vi "EEG read with Filtered PSD Features and classifier with Wii BB FINAL DEMO VERSION.vi"() -> ()   [LabVIEW 2010]
uses:
  <vilib>/Analysis/4window.llb/windowTd.ctl
  <vilib>/Utility/error.llb/DialogType.ctl
  <vilib>/Platform/TimedLoop/XDataNode/XDataNode.xnode
  <vilib>/Platform/TimedLoop/XDataNode/timing_clust.ctl
  <vilib>/Platform/TimedLoop/XDataNode/nitl_modes.ctl
  <vilib>/Platform/TimedLoop/XDataNode/wakeup.ctl
  <vilib>/measure/maspectr.llb/Power Spectrum and PSD Export Mode.ctl
  <vilib>/Analysis/3filter.llb/Filter Passband Type.ctl
  <vilib>/DAQmx/read.llb/DAQmx Read (Analog Wfm 1Chan NSamp).vi
  <vilib>/DAQmx/create/channels.llb/DAQmx Create Channel (AI-Voltage-Basic).vi
  <vilib>/DAQmx/configure/timing.llb/DAQmx Timing (Sample Clock).vi
  <vilib>/Utility/file.llb/Write To Spreadsheet File (DBL).vi
  <vilib>/Analysis/3filter.llb/Butterworth Filter (DBL).vi
  <vilib>/measure/matone.llb/Extract Single Tone Information 1 Chan.vi
  <vilib>/measure/maspectr.llb/FFT Power Spectrum and PSD for 1 Chan.vi
  <vilib>/daqmx/miscellaneous.llb/DAQmx Fill In Error Info.vi
  <vilib>/Waveform/WDTFileIO.llb/Export Waveform To Spreadsheet File.vi
  <vilib>/measure/NI_MAPro.lvlib
  <vilib>/Analysis/NI_AALBase.lvlib
  <vilib>/Analysis/NI_AAL_SigProc.lvlib
  <vilib>/Platform/TimedLoop/XDataNode/XDNodeRunTimeDep.lvlib
  <vilib>/Analysis/NI_AALPro.lvlib
panel:
  in  "input terminal configuration":i32(ring)=-1 items=["default"=-1, "RSE"=10083, "NRSE"=10078, "Differential"=10106, "Pseudodifferential"=12529]
  in  "Save Wii BB":bool
  in  "stop 2":bool
  in  "index":i32
  out "Button":bool
  out "X":dbl
  out "Y":dbl
  in  "LED":bool
  out "error out":errorcluster
  out "XY Balance Board":cluster{dbl[], dbl[]}(graph)
  in  "Low Cutoff Frequency":dbl(slide) scale=0.0..100.0
  in  "High Cutoff Frequency":dbl(slide) scale=0.0..500.0
  in  "String to be appended in filename":string
  in  "Slide":dbl(slide) scale=0.0..0.0005
  in  "WINDOW":T1=1 items=["Rectangle"=0, "Hanning"=1, "Hamming"=2, "Blackman-Harris"=3, "Exact Blackman"=4, "Blackman"=5, "Flat Top"=6, "4 Term B-Harris "=7, "7 Term B-Harris"=8, "Low Sidelobe"=9, "Blackman Nuttall"=11, "Triangle"=30, "Bartlett-Hanning"=31, "Bohman"=32, "Parzen"=33, "Welch"=34, "Kaiser"=60, "Dolph-Chebyshev"=61, "Gaussian"=62]
  out "Amplitudes":dbl[](array[numeric])
  out "FREQUENCY":dbl[](array[numeric])
  in  "Min. No. of Peaks\n to be detected":i32
  out "# found":i32
  out "BRAIN SWITCH":bool
  out "PSD Filtered Waveform":cluster{"f0":dbl, "df":dbl, "magnitude":dbl[]}(graph)
  in  "Path":path
  in  "SAVE TO FILE":bool
  out "new file path (Not A Path if cancelled)":path
  out "df":dbl
  out "magnitude":dbl[](array[numeric])
  out "f0":dbl
  in  "PARAMETERS":T2={"averaging mode"=enum."No averaging", "weighting mode"=enum."Linear", "number of averages"=10}
  out "Test SIGNAL AMPLITUDE":dbl format="%.2p"
  out "Test SIGNAL FREQUENCY":dbl format="%.2p"
  in  "BUFFER SIZE":dbl
  out "FILTERED Waveform Graph":waveform(dbl)(graph)
  in  "stop":bool
  in  "SAMPLE RATE":dbl=1000.0 format="%0.2f"
  # "EEG DATA ACQUISITION AND ANALYSIS"
  # "DAQ PARAMETERS"
  # "FEATURES EXTRACTED"
  # "BAND PASS FILTER CHARACTERSTICS"
  # "AVERAGING PARAMETERS and FEATURES EXTRACTED FROM THE FILTERED PSD"
  # "Wii BB CONTROLS and INDICATORS"
  # "THRESHOLD CLASSIFIER"
  # "FILE SAVING MODULE"
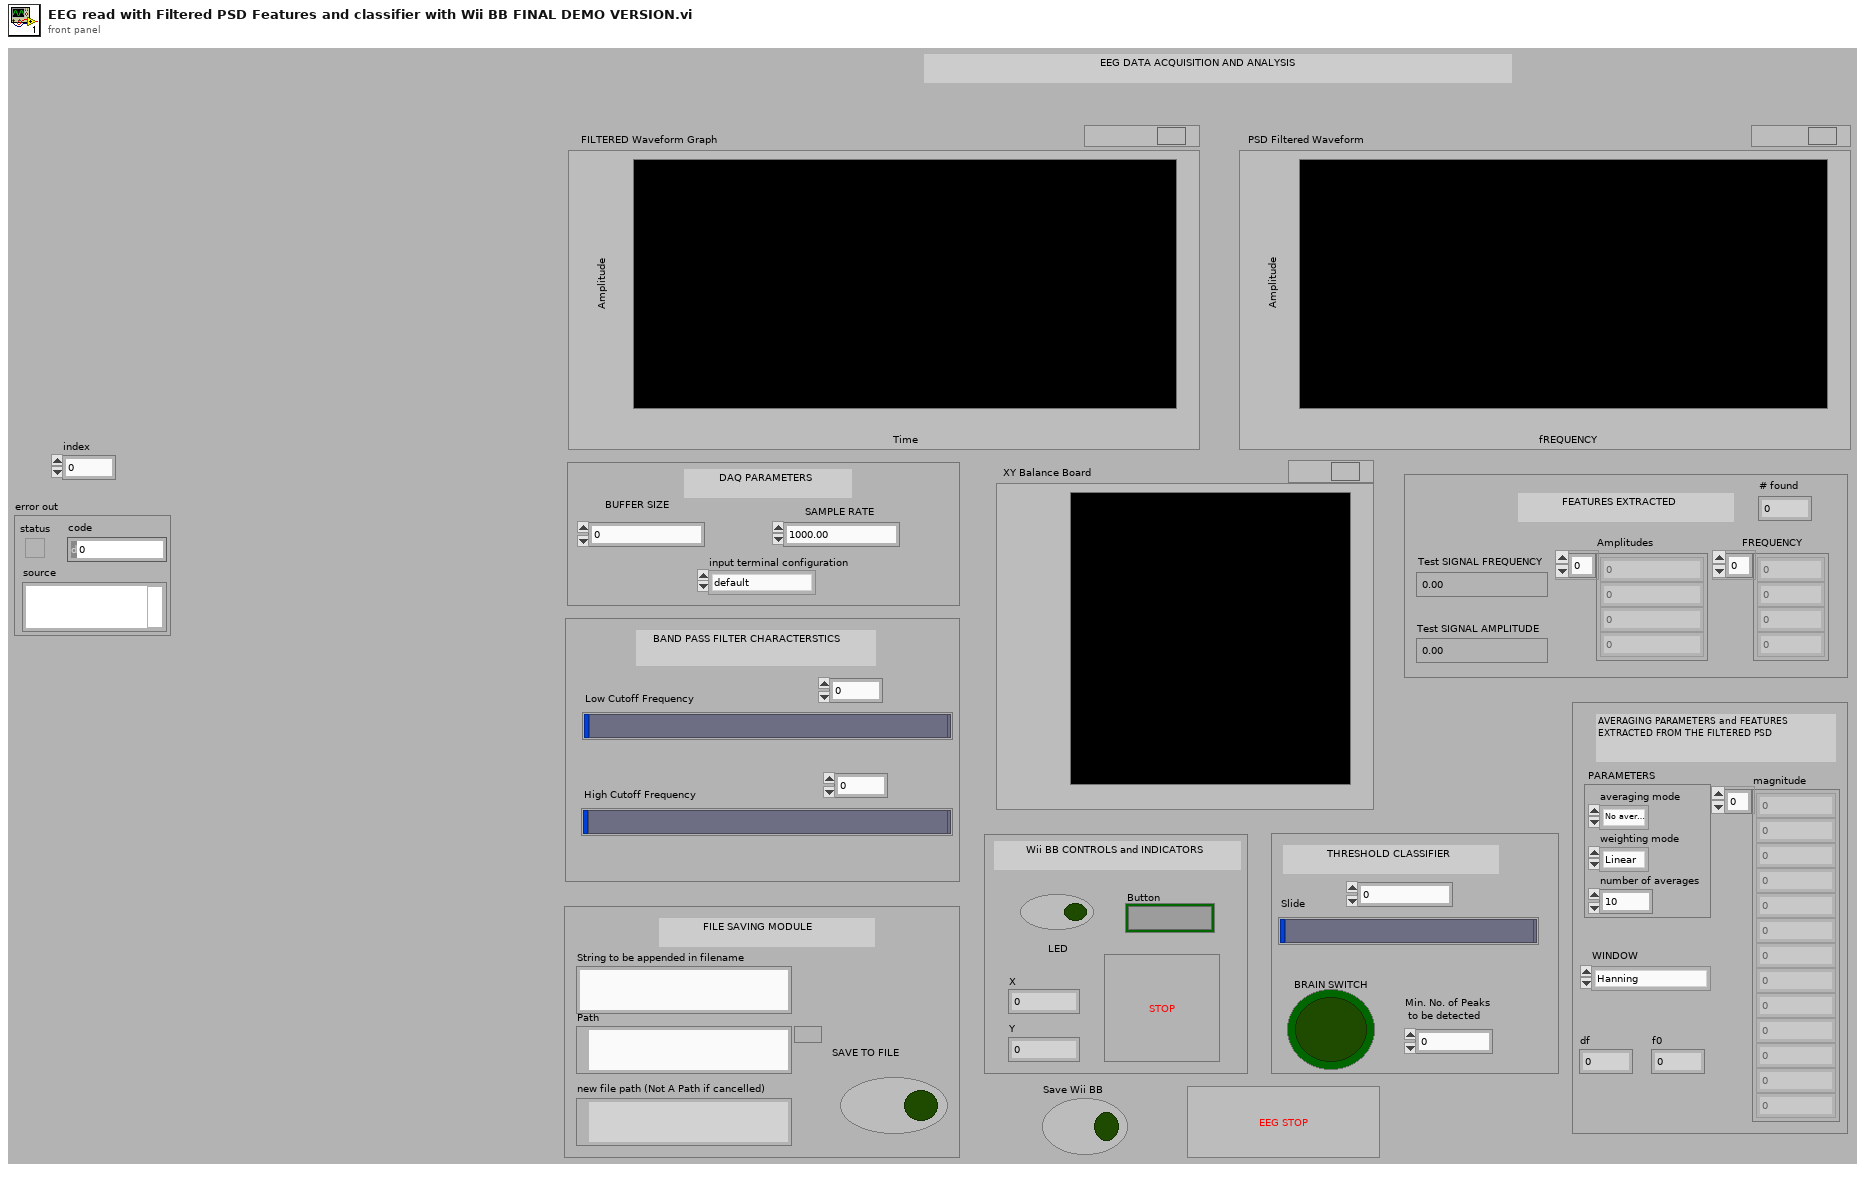
[diagram p1: front panel]
types:
  T1 = typedef "NI_AALPro.lvlib/windowTd.ctl" = u32
  T2 = cluster{"averaging mode":enum16{"No averaging", "Vector averaging", "RMS averaging", "Peak hold"}, "weighting mode":enum16{"Linear", "Exponential"}, "number of averages":u32}
  T3 = typedef "DialogType.ctl" = u16
  T4 = cluster{"right-top zero":i16, "right-bottom zero":i16, "left-top zero":i16, "left-bottom zero":i16}
  T5 = cluster{"Right-top":i16, "Right-bottom":i16, "Left-top":i16, "Left-bottom":i16, "X":dbl, "Y":dbl, "Sum":dbl}
  T6 = typedef "NI_Matrix.lvlib/RealMatrix.ctl" = dbl[][]
  T7 = typedef "XDNodeRunTimeDep.lvlib/timing_clust.ctl" = cluster{"Expected End [f-1]":u64, "Actual End [f-1]":u64, "Finished Late? [f-1]":bool, "Expected End [i-1]":u64, "Actual End [i-1]":u64, "Finished Late? [i-1]":bool, "Expected Start [i]":u64, "Actual Start [i]":u64, "Expected Start [f]":u64, "Actual Start [f]":u64, "Source Name":string, "Structure Name":string, "Period":i64, "Deadline":i64, "Offset":i64, "Start":i64, "Priority":i32, "Timeout":i32, "Mode":T8, "Wakeup Reason":T9, "Error":errorcluster, "Source Type":string, "Secondary Source Type":string, "Global End Time":u64, "Global Start Time":u64, "Frame Duration":u64, "Iteration Duration":u64, "Assigned CPU":i32, "I/O Scan Engine Mode":u32}
  T8 = typedef "XDNodeRunTimeDep.lvlib/nitl_modes.ctl" = enum32{"No Change", "Process missed periods, maintain original phase", "Discard missed periods, maintain original phase", "Process missed periods, ignore original phase", "Discard missed periods, ignore original phase"}
  T9 = typedef "XDNodeRunTimeDep.lvlib/wakeup.ctl" = enum32{"Normal", "Aborted", "Asynchronous wakeup", "Timing source error", "Timed loop error", "Timeout"}
  T10 = typedef "NI_AALBase.lvlib/Filter Passband Type.ctl" = enum32{"Lowpass", "Highpass", "Bandpass", "Bandstop"}
  T11 = typedef "NI_MAPro.lvlib/Power Spectrum and PSD Export Mode.ctl" = u16
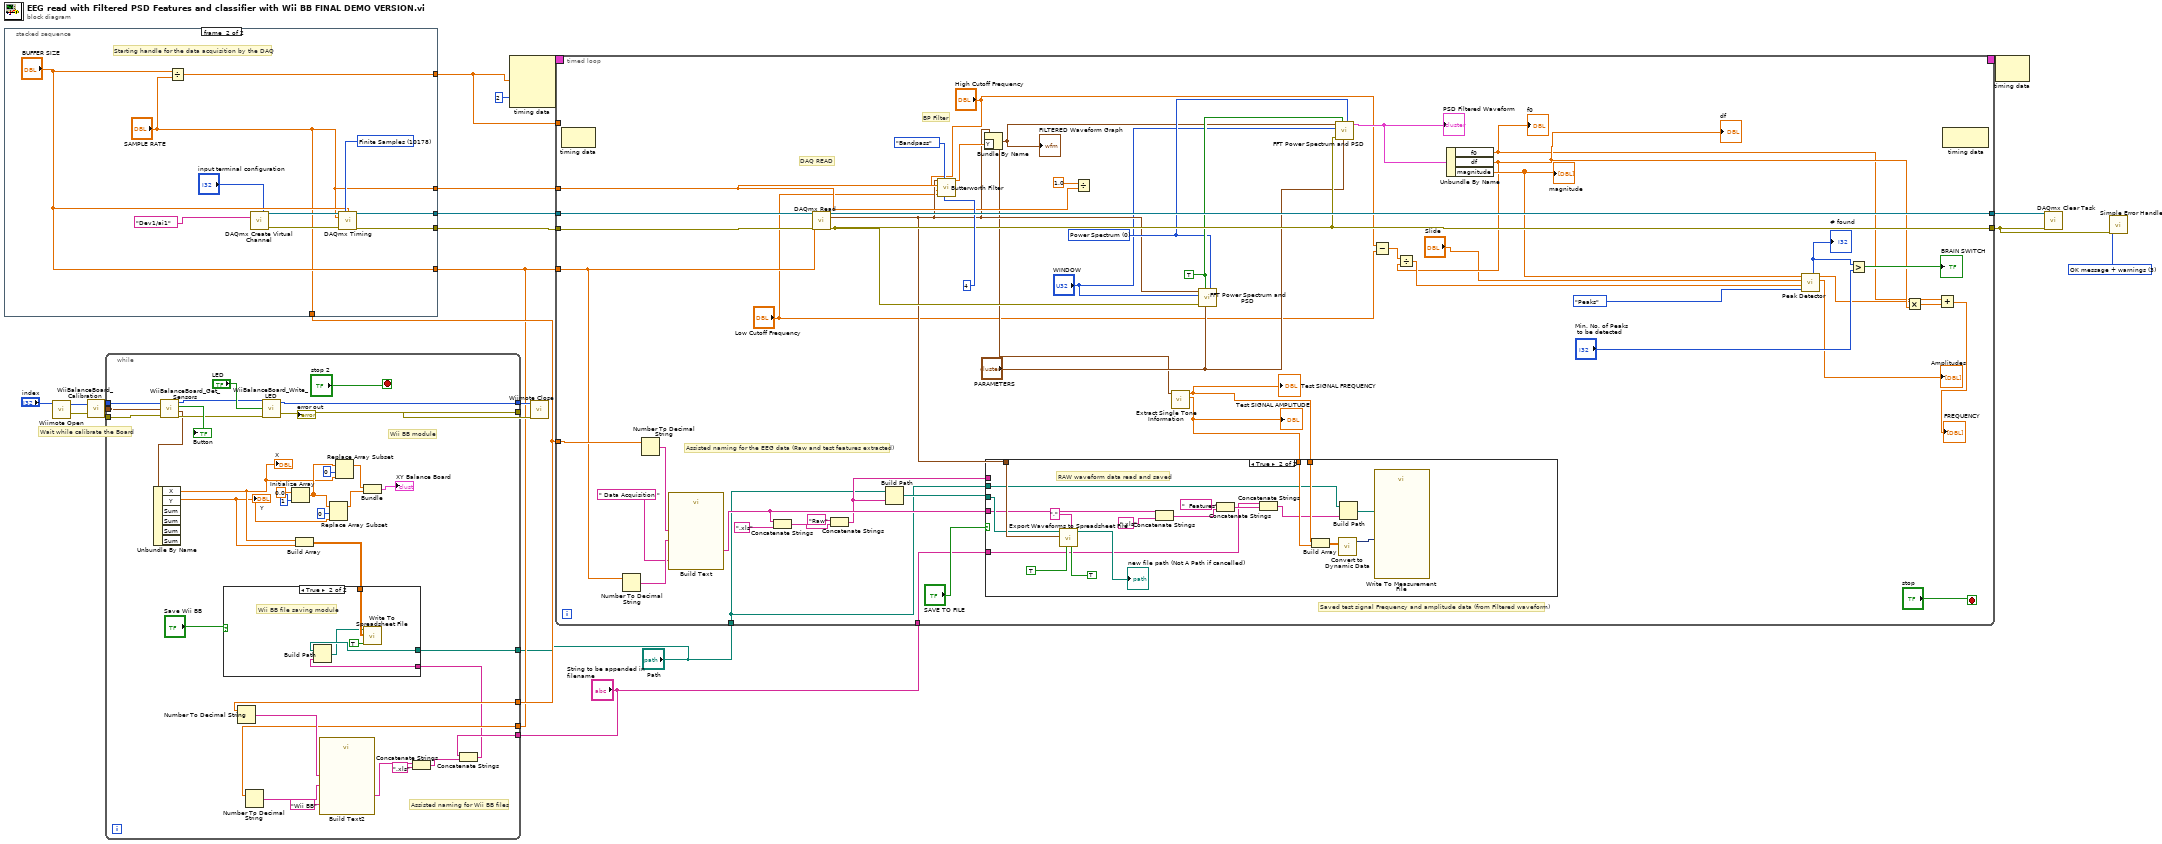
[diagram p0: block diagram]
diagram:
  w14 = T3 3 items=["no dialog", "OK message", "continue or stop message", "OK message + warnings", "continue/stop + warnings"] ("type of dialog (OK msg:1)")
  # "Wait while calibrate the Board"
  n1 = stacked-sequence {
    tunnel: [_ "SAMPLE RATE"] -> w19
    tunnel: [_ "BUFFER SIZE"] -> w3
    tunnel: [_ w27] -> w18
    tunnel: [_ w26] -> w17
    tunnel: [_ w25] -> w5
    tunnel: [_ "SAMPLE RATE"] -> w4
    frame #0 {
    }
    frame #1 {
      w31 = 10178 items=["Finite Samples"=10178, "Continuous Samples"=10123, "Hardware Timed Single Point"=12522] ("sample mode")
      # "Starting handle for the data acquisition by the DAQ"
      n2 = Divide(x="BUFFER SIZE", y="SAMPLE RATE") -> (x/y=w25:dbl)
      n3 = call-poly <vilib>:"DAQmx Create Virtual Channel.vi"("input terminal configuration"="input terminal configuration", "physical channels"=tag "Dev1/ai1") -> ("task out"=w29:refnum<k21>, "error out"=w30:errorcluster)  [unwired: 12 in]
      n4 = call-poly <vilib>:"DAQmx Timing.vi"("task/channels in"=w29, "sample mode"=w31, "samples per channel"="BUFFER SIZE", "rate"="SAMPLE RATE", "error in"=w30) -> ("task out"=w27:refnum<k21>, "error out"=w26:errorcluster)  [unwired: 9 in]
    }
  }
  n5 = call "Wiimote Open.vi"("index"="index") -> ("error out"=w9:errorcluster, "hWiimoteHandle"=w10:u32)  [unwired: 9 in]
  n6 = call "WiiBalanceBoard_Calibration.vi"("hWiimoteHandle in"=w10, "error in"=w9) -> ("hWiimoteHandle out"=w8:u32, "Wii Balance Board Zeros"=w6:T4, "error out"=w7:errorcluster)
  n7 = while {
    tunnel: [w64] -> w12
    tunnel: [w63] -> w11
    tunnel: w8 -> [w60]
    tunnel: w7 -> [w59]
    tunnel: w6 -> [w58]
    tunnel: w4 -> [w43]
    tunnel: w3 -> [w41]
    tunnel: "String to be appended in filename" -> [w36]
    tunnel: "Path" -> [w33]
    stop <- "stop 2" stop-if-true
    # "Assisted naming for Wii BB files"
    # "Wii BB module"
    n8 = call "WiiBalanceBoard_Get_Sensors.vi"("hWiimoteHandle in"=w60, "Wii Balance Board Zeros"=w58, "error in"=w59) -> ("hWiimoteHandle out"=w51:u32, "Button"=→"Button":bool, "Wii Balance Board Sensors"=w49:T5, "error out"=w50:errorcluster)  [unwired: 1 out]
    n9 = Unbundle By Name(w49) -> ("X"=w47:dbl, "Y"=w46:dbl)  [unwired: 4 out]
    "X" <- w47
    "Y" <- w46
    n10 = Number To Decimal String(number=w43) -> (decimal integer string=w42:string)  [unwired: 1 in]
    n11 = Number To Decimal String(number=w41) -> (decimal integer string=w40:string)  [unwired: 1 in]
    n12 = call "WiiBalanceBoard_Write_LED.vi"("error in"=w50, "Balance Board LED"="LED", "hWiimoteHandle in"=w51) -> ("error out"=w63:errorcluster, "hWiimoteHandle out"=w64:u32)
    "error out" <- w63
    n13 = Initialize Array(0.0 ("element"), 1 ("dimension size")) -> (w53:dbl[])
    n14 = Build Array(w47, w46) -> (w45:T6)
    n15 = call "Build Text2"("Beginning Text"="Wii BB", "Frequency"=w42, "Buffer"=w40) -> ("Result"=w38:string)  [unwired: 11 in, 1 out]
    n16 = Replace Array Subset(array=w53, new element=w46, index=0) -> (w61:dbl[])
    n17 = Replace Array Subset(array=w53, new element=w47, index=0) -> (w62:dbl[])
    n18 = Bundle(w62, w61) -> (→"XY Balance Board":cluster{dbl[], dbl[]})  [unwired: 1 in]
    n19 = Concatenate Strings(w38, ".xls" ("string")) -> (w35:string)
    n20 = Concatenate Strings(w36, w35) -> (w34:string)
    n21 = case shown="True" "Save Wii BB" {
      tunnel: w45 -> [_ w71]
      tunnel: w34 -> [_ w69]
      tunnel: w33 -> [_ w68]
      frame False {
      }
      frame True {
        # "Wii BB file saving module"
        n22 = Build Path(base path=w68, name or relative path=w69) -> (appended path=w67:path)
        n23 = call-poly <vilib>:"Write To Spreadsheet File.vi"("append to file? (new file:F)"=TRUE, "2D data"=w71, "file path (dialog if empty)"=w67) -> ()  [unwired: 5 in, 1 out]
      }
    }
  }
  n24 = node-c288(w5, 2 ("Processor")) -> (w22:T7)  [unwired: 2 in]
  n25 = call "Wiimote Close.vi"("error in"=w11, "hWiimoteHandle in"=w12) -> ()  [unwired: 9 in, 1 out]
  n26 = timed-loop {
    timing: w22 -> [_]
    timing-out: [_] -> w21
    tunnel: w18 -> [w118]
    tunnel: w17 -> [w119]
    tunnel: [w104] -> w15
    tunnel: [w117] -> w20
    tunnel: w19 -> [w113]
    tunnel: w3 -> [w108]
    tunnel: w5 -> [_]
    tunnel: w4 -> [w110]
    tunnel: "String to be appended in filename" -> [w73]
    tunnel: "Path" -> [w72]
    stop <- "stop" stop-if-true
    w103 = TRUE ("restart averaging (F)")
    w102 = T11 0 items=["Power Spectrum", "Power Spectral Density"] ("export mode")
    # "Saved test signal Frequency and amplitude data (from Filtered waveform)"
    # "BP Filter"
    # "DAQ READ"
    # "Assisted naming for the EEG data (Raw and test features extracted)"
    n27 = node-c288() -> ()  [unwired: 1 in, 1 out]
    n28 = Number To Decimal String(number=w108) -> (decimal integer string=w107:string)  [unwired: 1 in]
    n29 = Number To Decimal String(number=w110) -> (decimal integer string=w109:string)  [unwired: 1 in]
    n30 = call "Build Text"("Beginning Text"=" Data Acquisition ", "Frequency"=w109, "Buffer"=w107) -> ("Result"=w99:string)  [unwired: 11 in, 1 out]
    n31 = Concatenate Strings(w99, ".xls" ("string")) -> (w97:string)
    n32 = call-poly <vilib>:"DAQmx Read.vi"("task/channels in"=w118, "number of samples per channel"=w108, "error in"=w119) -> ("task out"=w117:refnum<k21>, "data"=w95:waveform(dbl), "error out"=w104:errorcluster)  [unwired: 10 in]
    n33 = Concatenate Strings("Raw" ("string"), w97) -> (w96:string)
    n34 = Build Path(base path=w72, name or relative path=w96) -> (appended path=w111:path)
    n35 = call-poly <vilib>:"Butterworth Filter.vi"("order"=4, "filter type"=Filter_Passband_Type."Bandpass", "low cutoff freq: fl"="Low Cutoff Frequency", "high cutoff freq: fh"="High Cutoff Frequency", "sampling freq: fs"=w113, "X"=w95) -> ("Filtered X"=w100:dbl[])  [unwired: 2 in, 1 out]
    n36 = Bundle By Name(cluster=w95, "Y"=w100) -> (w76:waveform(dbl))
    "FILTERED Waveform Graph" <- w76
    n37 = Divide(x=1.0, y=w113) -> ()  [unwired: 1 out]
    n38 = call-poly <vilib>:"Extract Single Tone Information.vi"("time signal in"=w76) -> ("detected amplitude"=w94:dbl, "detected frequency"=w80:dbl)  [unwired: 5 in, 4 out]
    "Test SIGNAL FREQUENCY" <- w80
    "Test SIGNAL AMPLITUDE" <- w94
    n39 = case shown="True" "SAVE TO FILE" {
      tunnel: w95 -> [_ w139]
      tunnel: w111 -> [_ w132]
      tunnel: w80 -> [_ w134]
      tunnel: w94 -> [_ w126]
      tunnel: w96 -> [_ _]
      tunnel: w99 -> [_ w124]
      tunnel: w72 -> [_ w125]
      tunnel: w73 -> [_ w121]
      frame False {
      }
      frame True {
        # "RAW waveform data read and saved"
        n40 = call-poly <vilib>:"Export Waveforms to Spreadsheet File.vi"("header? (write header:T)"=TRUE, "delimiter (Tab)"=",", "append to file? (new file:F)"=TRUE, "waveform"=w139, "file path (dialog if empty)"=w132) -> ("new file path (Not A Path if cancelled)"=→"new file path (Not A Path if cancelled)":path)  [unwired: 5 in, 1 out]
        n41 = Concatenate Strings(w124, ".xls" ("string")) -> (w128:string)
        n42 = Concatenate Strings("  Features" ("string"), w128) -> (w122:string)
        n43 = Concatenate Strings(w121, w122) -> (w123:string)
        n44 = Build Array(w134, w126) -> (w133:T6)
        n45 = call "Convert to Dynamic Data"("2D Array"=w133) -> ("Dynamic Data Type"=w135:dynamicdata)  [unwired: 3 in]
        n46 = Build Path(base path=w125, name or relative path=w123) -> (appended path=w130:path)
        n47 = call "Write To Measurement File"("Signals"=w135, "Filename"=w130) -> ()  [unwired: 15 in, 3 out]
      }
    }
    n48 = call-poly <vilib>:"FFT Power Spectrum and PSD.vi"("export mode"=w102, "averaging parameters"="PARAMETERS", "restart averaging (F)"=w103, "error in (no error)"=w104, "window"="WINDOW", "time signal"=w95) -> ()  [unwired: 2 in, 4 out]
    n49 = call-poly <vilib>:"FFT Power Spectrum and PSD.vi"("export mode"=w102, "averaging parameters"="PARAMETERS", "restart averaging (F)"=w103, "error in (no error)"=w104, "window"="WINDOW", "time signal"=w76) -> ("Power Spectrum / PSD"=w93:cluster{"f0":dbl, "df":dbl, "magnitude":dbl[]})  [unwired: 2 in, 3 out]
    "PSD Filtered Waveform" <- w93
    n50 = Subtract(x="High Cutoff Frequency", y="Low Cutoff Frequency") -> (x-y=w91:dbl)
    n51 = Unbundle By Name(w93) -> ("f0"=w84:dbl, "df"=w85:dbl, "magnitude"=w92:dbl[])
    "f0" <- w84
    "magnitude" <- w92
    "df" <- w85
    n52 = Divide(x=w91, y=w85) -> (x/y=w90:dbl)
    n53 = call <vilib>:"Peak Detector.vi"("peaks/valleys"=enum32{"Peaks", "Valleys"}."Peaks", "width"=w90, "threshold"="Slide", "X"=w92) -> ("Amplitudes"=→"Amplitudes":dbl[], "Locations"=w83:dbl[], "# found"=w88:i32)  [unwired: 3 in, 2 out]
    "# found" <- w88
    n54 = Greater?(x=w88, y="Min. No. of Peaks\n to be detected") -> (0:→"BRAIN SWITCH":bool)
    n55 = Multiply(x=w83, y=w85) -> (x*y=w82:dbl[])
    n56 = Add(x=w84, y=w82) -> (x+y=→"FREQUENCY":dbl[])
    n57 = node-c288() -> ()  [unwired: 1 in, 1 out]
  }
  n58 = node-c288(w21) -> ()  [unwired: 1 out]
  n59 = call <vilib>:"DAQmx Clear Task.vi"("task in"=w20, "error in"=w15) -> ()  [unwired: 13 in, 1 out]
  n60 = call <vilib>:"Simple Error Handler.vi"("type of dialog (OK msg:1)"=w14, "error in (no error)"=w15) -> ()  [unwired: 3 in, 5 out]
